vi "Log.vi"(7 "Event Level":T1, 8 "error in (no error)":errorcluster, 10 "Data To Log":string, 11 "SessionHandler in":refnum<class "SessionHandler.lvclass">) -> (0 "error out":errorcluster, 3 "SessionHandler out":refnum<class "SessionHandler.lvclass">)   [LabVIEW 2019, in "Network Sink.lvlib" / "SessionHandler.lvclass"]
uses:
  <vilib>/gpm_packages/@cs/event-logger/Source/Network Sink/SessionHandler/SessionHandler.lvclass
  <vilib>/gpm_packages/@cs/event-logger/Source/Composed Log/Types/Log Level.ctl
  <vilib>/gpm_packages/@cs/event-logger/Source/Network Sink/SessionHandler/SessionHandler.lvclass/SessionHandler.ctl
  <vilib>/gpm_packages/@cs/event-logger/Source/Composed Log/LoggerReference/LoggerReference.lvclass/LoggerReference.ctl
  <vilib>/gpm_packages/@cs/event-logger/Source/Composed Log/LoggerReference/Get Valid Event Time.vi
  <vilib>/gpm_packages/@cs/event-logger/Source/Composed Log/LoggerReference/Remove Stale Logs.vi
  <vilib>/gpm_packages/@cs/event-logger/Source/Composed Log/LoggerReference/LoggerReference.lvclass
  <vilib>/gpm_packages/@cs/event-logger/Source/Composed Log/Composed Log.lvlib
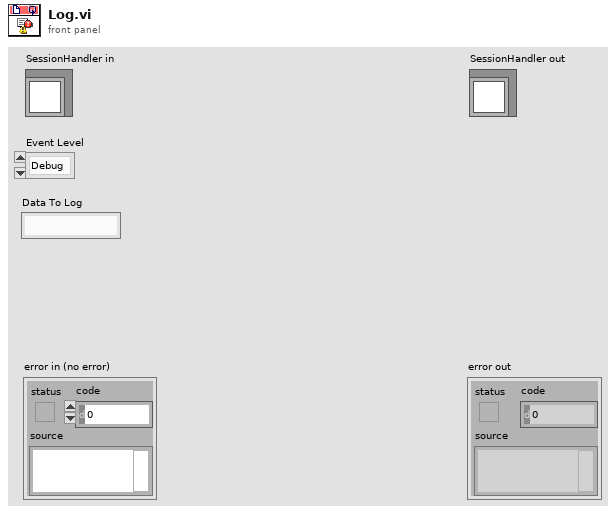
[diagram p1: front panel]
types:
  T1 = typedef "Composed Log.lvlib/Log Level.ctl" = enum16{"Debug", "Info", "Warning", "Error", "Critical"}
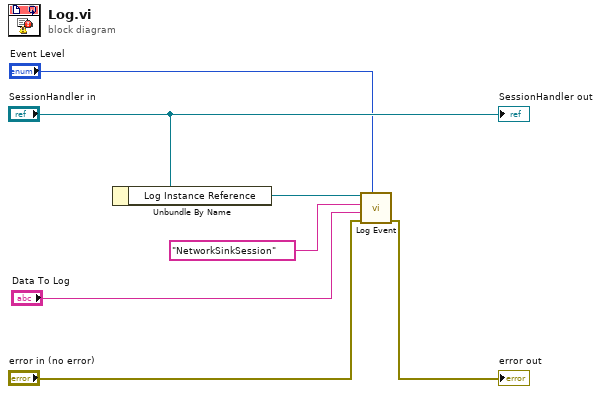
[diagram p0: block diagram]
diagram:
  n1 = Unbundle By Name("SessionHandler in") -> ("Log Instance Reference"=w6:refnum<class "LoggerReference.lvclass">)
  n2 = call <vilib>:"Log Event.vi"("Event Level"="Event Level", "error in (no error)"="error in (no error)", "Data To Log"="Data To Log", "SourceID"="NetworkSinkSession", "Log Instance"=w6) -> ("error out"=→"error out":errorcluster)  [unwired: 5 in, 1 out]
  "SessionHandler out" <- "SessionHandler in"
